vi "initialize.vi"(8 "error in (no error)":errorcluster, 11 "SwitchBoxConrad in":refnum<class "SwitchBoxConrad.lvclass">) -> (0 "error out":errorcluster, 1 "String outout":string, 2 "initialized?":bool, 3 "SwitchBoxConrad out":refnum<class "SwitchBoxConrad.lvclass">)   [LabVIEW 2018, in "SwitchBoxConrad.lvclass"]
doc: "initializes an instrument; this method is going to be replaced by the same method of the child objects"
uses:
  SwitchBoxConrad.lvclass
  fddb8e39-4018-420b-b964-ebf1ced4499d.vi
  instrument.lvclass
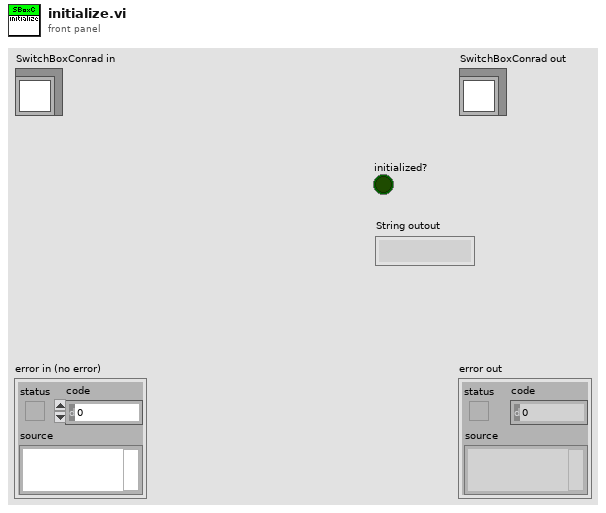
[diagram p1: front panel]
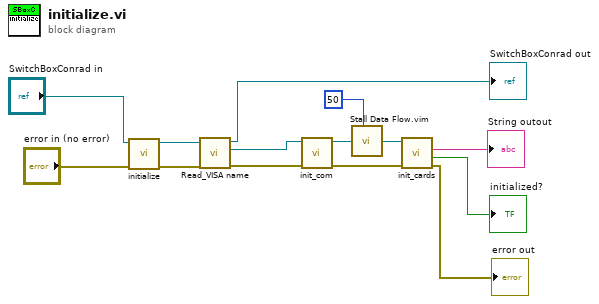
[diagram p0: block diagram]
diagram:
  n1 = call-parent "initialize.vi"("error in (no error)"="error in (no error)", "instrument in"="SwitchBoxConrad in") -> ("error out"=w11:errorcluster, "instrument out"=w12:refnum<class "SwitchBoxConrad.lvclass">)  [unwired: 6 in, 2 out]
  n2 = call-dynamic "Read_VISA name.vi"("error in (no error)"=w11, "instrument in"=w12) -> ("error out"=w9:errorcluster, "VISA resource name"=w10:refnum<visa-resource-name>, "instrument out"=→"SwitchBoxConrad out":refnum<class "SwitchBoxConrad.lvclass">)  [unwired: 7 in]
  n3 = call "init_com.vi"("error in (no error)"=w9, "VISA Refnum in"=w10) -> ("error out"=w8:errorcluster, "VISA Refnum out"=w3:refnum<visa-resource-name>)  [unwired: 8 in]
  n4 = call "Stall Data Flow.vim"("value in"=w3, "milliseconds to wait"=u32 50) -> ("value out"=w2:refnum<visa-resource-name>)  [unwired: 1 out]
  n5 = call "init_cards.vi"("error in (no error)"=w8, "VISA Refnum in"=w2) -> ("error out"=→"error out":errorcluster, "init ok?"=→"initialized?":bool, "read buffer"=→"String outout":string)  [unwired: 6 in, 1 out]
